vi "Excute.vi"(8 "error in (no error)":errorcluster, 11 "Base in":refnum<class "Base.lvclass">) -> (0 "error out":errorcluster, 3 "Base out":refnum<class "Base.lvclass">)   [LabVIEW 2014, in "Framework.lvlib" / "Base.lvclass"]
uses:
  Base.lvclass
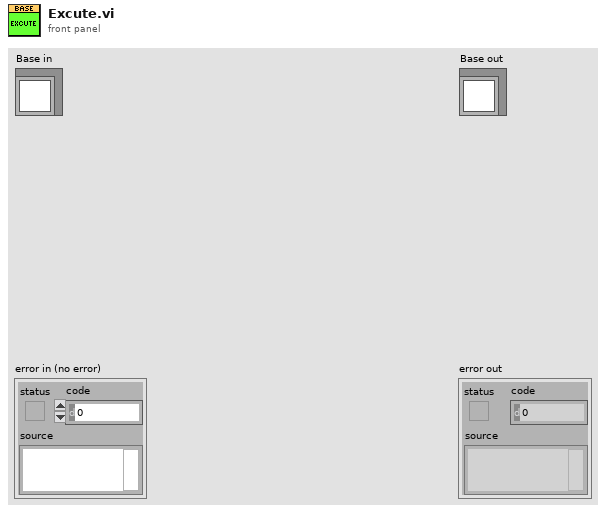
[diagram p1: front panel]
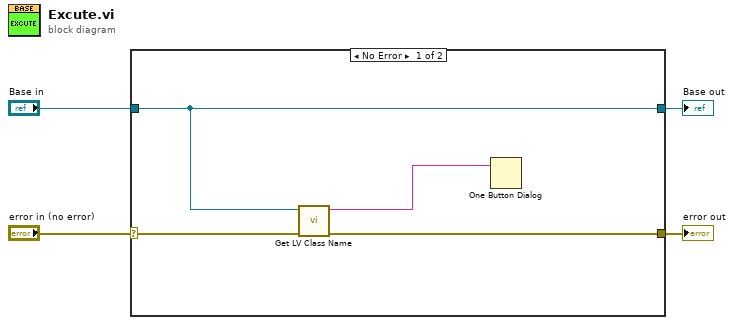
[diagram p0: block diagram]
diagram:
  n1 = case shown="No Error" "error in (no error)" {
    selector: "error in (no error)" -> [w6 w10]
    tunnel: [w5 w10] -> w3
    tunnel: [w8 w9] -> w1
    tunnel: "Base in" -> [w8 w9]
    frame No Error {
      n2 = call <vilib>:"Get LV Class Name.vi"("error in (no error)"=w6, "object"=w8) -> ("error out"=w5:errorcluster, "class name"=w7:string)  [unwired: 8 in]
      n3 = One Button Dialog(message=w7) -> ()  [unwired: 1 in, 1 out]
    }
    frame Error {
    }
  }
  "error out" <- w3
  "Base out" <- w1
